vi "FileWriteTest.vi"() -> ()   [LabVIEW 2017]
uses:
  <vilib>/Utility/sysdir.llb/System Directory Type.ctl
panel:
  out "Seconds":i32
  in  "stop":bool
  out "File Name":string
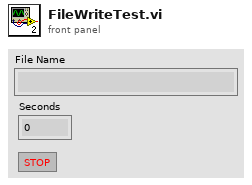
[diagram p1: front panel]
types:
  T1 = enum16{"open", "replace", "create", "open or create", "replace or create", "replace or create with confirmation"}
  T2 = typedef "System Directory Type.ctl" = i32
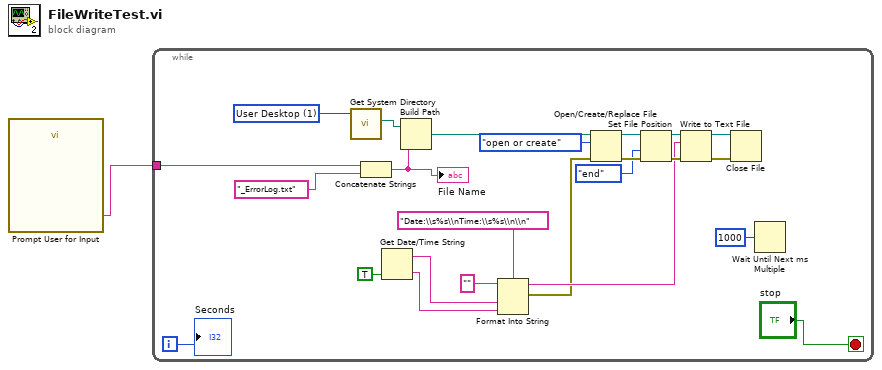
[diagram p0: block diagram]
diagram:
  n1 = call "Prompt User for Input"() -> ("File Name"=w1:string)  [unwired: 17 in, 2 out]
  n2 = while {
    tunnel: w1 -> [w4]
    i -> [w8]
    stop <- "stop" stop-if-true
    w16 = T2 1 items=["User Home"=0, "User Desktop"=1, "User Documents"=2, "User Application Data"=3, "User Preferences"=4, "User Temporary"=5, "Public Documents"=6, "Public Application Data"=7, "Public Preferences"=8, "Public Cache"=13, "System Core Libraries"=9, "System Installed Libraries"=10, "Application Files"=11, "Boot Volume Root"=12] ("system directory type")
    n3 = call <vilib>:"Get System Directory.vi"("system directory type"=w16) -> ("system directory"=w25:path)  [unwired: 10 in]
    n4 = Concatenate Strings(w4, "_ErrorLog.txt" ("name or relative path")) -> (w2:string)
    "File Name" <- w2
    n5 = Get Date/Time String(want seconds? (F)=TRUE) -> (date string=w6:string, time string=w7:string)  [unwired: 2 in]
    n6 = Build Path(base path=w25, name or relative path=w2) -> (appended path=w3:path)
    n7 = Format Into String(format string="Date:\\s%s\\nTime:\\s%s\\n\\n", initial string="" ("input 2"), w6, w7) -> (resulting string=w13:string, error out=w9:errorcluster)  [unwired: 1 in]
    n8 = Open/Create/Replace File(file path (use dialog)=w3, error in=w9, operation (0:open)=T1."open or create") -> (refnum out=w22:refnum<file>, error out=w23:errorcluster)  [unwired: 3 in, 1 out]
    n9 = Set File Position(refnum=w22, from (0:start)=enum16{"start", "end", "current"}."end", error in=w23) -> (refnum out=w18:refnum<file>, error out=w21:errorcluster)  [unwired: 1 in]
    n10 = Write to Text File(file (use dialog)=w18, text=w13, error in=w21) -> (refnum out=w19:refnum<file>, error out=w20:errorcluster)  [unwired: 1 in, 1 out]
    n11 = Close File(refnum=w19, error in=w20) -> ()  [unwired: 2 out]
    n12 = Wait Until Next ms Multiple(millisecond multiple=u32 1000) -> ()  [unwired: 1 out]
    "Seconds" <- w8
  }
